vi "completed Write.vi"(4 "error in (no error)":errorcluster, 5 "Value":i32, 6 "Container State":T6, 7 "Display State In":T1={"Nspeakers"=13, "actions"=[], "Wspeaker"=13, "hover"={"type"=enum."None", "index"=0}, "locked"=FALSE, "states"=[], "sel speak"=13, "selected"=refnum, "Events"={"Selection change"=refnum}}) -> (0 "error out":errorcluster, 3 "Display State Out":T1={"Nspeakers"=13, "actions"=[], "Wspeaker"=13, "hover"={"type"=enum."None", "index"=0}, "locked"=FALSE, "states"=[], "sel speak"=13, "selected"=refnum, "Events"={"Selection change"=refnum}})   [LabVIEW 2015, in "SAC Config.xctl"]
uses:
  SAC Config.xctl
  <vilib>/_xctls/Container State.ctl
  State.vi
  Hover Data.ctl
  Hover Item.ctl
  Speaker State.ctl
  Events.ctl
  Selection changed.ctl
  <vilib>/_xctls/XControlSupport.lvlib
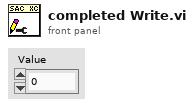
[diagram p1: front panel]
types:
  T1 = typedef "SAC Config.xctl/State.vi" = cluster{"Nspeakers":i32, "actions":string[], "Wspeaker":i32, "hover":T2, "locked":bool, "states":T4[], "sel speak":i32, "selected":refnum<vi>, "Events":T5}
  T2 = typedef "SAC Config.xctl/Hover Data.ctl" = cluster{"type":T3, "index":i32}
  T3 = typedef "SAC Config.xctl/Hover Item.ctl" = enum16{"None", "Speaker"}
  T4 = typedef "SAC Config.xctl/Speaker State.ctl" = cluster{"cal":bool, "selected":bool}
  T5 = typedef "SAC Config.xctl/Events.ctl" = cluster{"Selection change":refnum<user-event>}
  T6 = typedef "XControlSupport.lvlib/Container State.ctl" = cluster{"Indicator?":bool, "Run Mode?":bool, " Refnum":refnum<vi>}
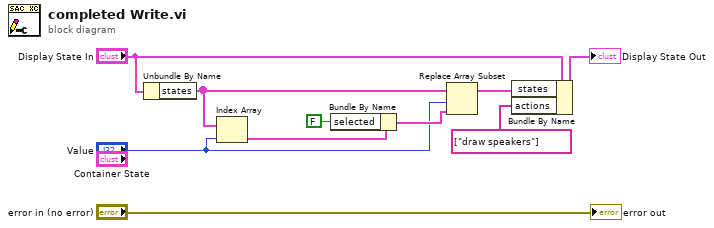
[diagram p0: block diagram]
diagram:
  n1 = Unbundle By Name("Display State In") -> ("states"=w5:T4[])
  n2 = Index Array(array=w5, index="Value") -> (element=w7:T4)
  n3 = Bundle By Name(cluster=w7, "selected"=FALSE) -> (w3:T4)
  n4 = Replace Array Subset(array=w5, new element=w3, index="Value") -> (w4:T4[])
  n5 = Bundle By Name(cluster="Display State In", "states"=w4, "actions"=string[] ["draw speakers"]) -> (→"Display State Out":T1)
  "error out" <- "error in (no error)"
